vi "ResetRunState.vi"(8 "error in (no error)":errorcluster, 11 "AutomationContext in":refnum<class "AutomationContext.lvclass">) -> (0 "error out":errorcluster, 3 "AutomationContext out":refnum<class "AutomationContext.lvclass">)   [LabVIEW 2023, in "Automation.lvlib" / "AutomationContext.lvclass"]
uses:
  AutomationContext.lvclass
  AutomationContext.lvclass/AutomationContext.ctl
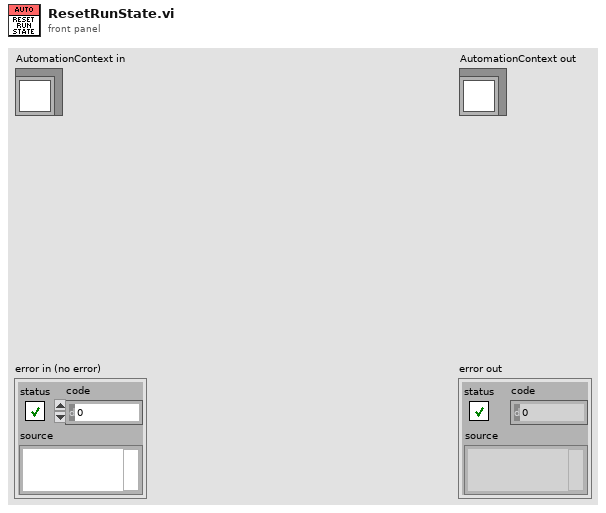
[diagram p1: front panel]
types:
  T1 = typedef "Automation.lvlib/AutomationContext.lvclass/Parallel Block.ctl" = cluster{"Tasks":T2[]}
  T2 = typedef "Automation.lvlib/AutomationContext.lvclass/Automation Intent.ctl" = cluster{"Action":T3, "Parameters":variant, "Correlation ID":u32}
  T3 = typedef "Automation.lvlib/AutomationContext.lvclass/Intent Action.ctl" = enum16{"Next Field", "Next Lane", "Set Power", "Reset Power", "Autofocus", "Start Streaming", "Delay", "Finish Run", "Open Shutter", "Close Shutter"}
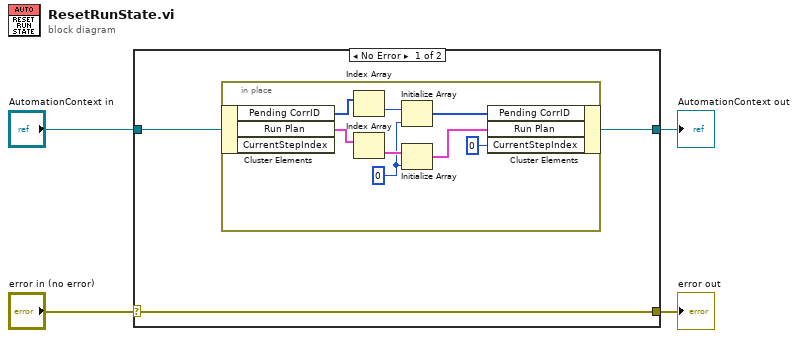
[diagram p0: block diagram]
diagram:
  n1 = case shown="No Error" "error in (no error)" {
    selector: "error in (no error)" -> [w7 w17]
    tunnel: [w7 w17] -> w3
    tunnel: [w5 w16] -> w1
    tunnel: "AutomationContext in" -> [w6 w16]
    frame No Error {
      n2 = in-place {
        w11 = 0 ("dimension size")
        n3 = in-place-cluster #1(w6) -> ("Pending CorrID"=w10:u32[], "Run Plan"=w14:T1[])  [unwired: 1 out]
        n4 = Index Array(array=w10) -> (element=w12:u32)  [unwired: 1 in]
        n5 = Index Array(array=w14) -> (element=w13:T1)  [unwired: 1 in]
        n6 = Initialize Array(w12, w11) -> (w9:u32[])
        n7 = Initialize Array(w13, w11) -> (w15:T1[])
        n8 = in-place-cluster #1("Pending CorrID"=w9, "Run Plan"=w15, "CurrentStepIndex"=u32 0) -> (w5:refnum<class "AutomationContext.lvclass">)
      }
    }
    frame Error {
    }
  }
  "error out" <- w3
  "AutomationContext out" <- w1
